vi "Test Control.vi"() -> ()   [LabVIEW 2012]
uses:
  2D Buffer Display.xctl
  <vilib>/Utility/miscctls.llb/LVBoundsTypeDef.ctl
  <vilib>/Utility/miscctls.llb/LVPositionTypeDef.ctl
panel:
  in  "Tab Control Pane Dimension":T1
  in  "Relative Size":dbl
  in  "Tab Control":enum32{"Page 1", "Page 2"}(tab)
  out "2D Buffer Display 3":cluster{"data_out":sgl[][], "time":timestamp}(xcontrol)
  out "2D Buffer Display 2":cluster{"data_out":sgl[][], "time":timestamp}(xcontrol)
  out "2D Buffer Display":cluster{"data_out":sgl[][], "time":timestamp}(xcontrol)
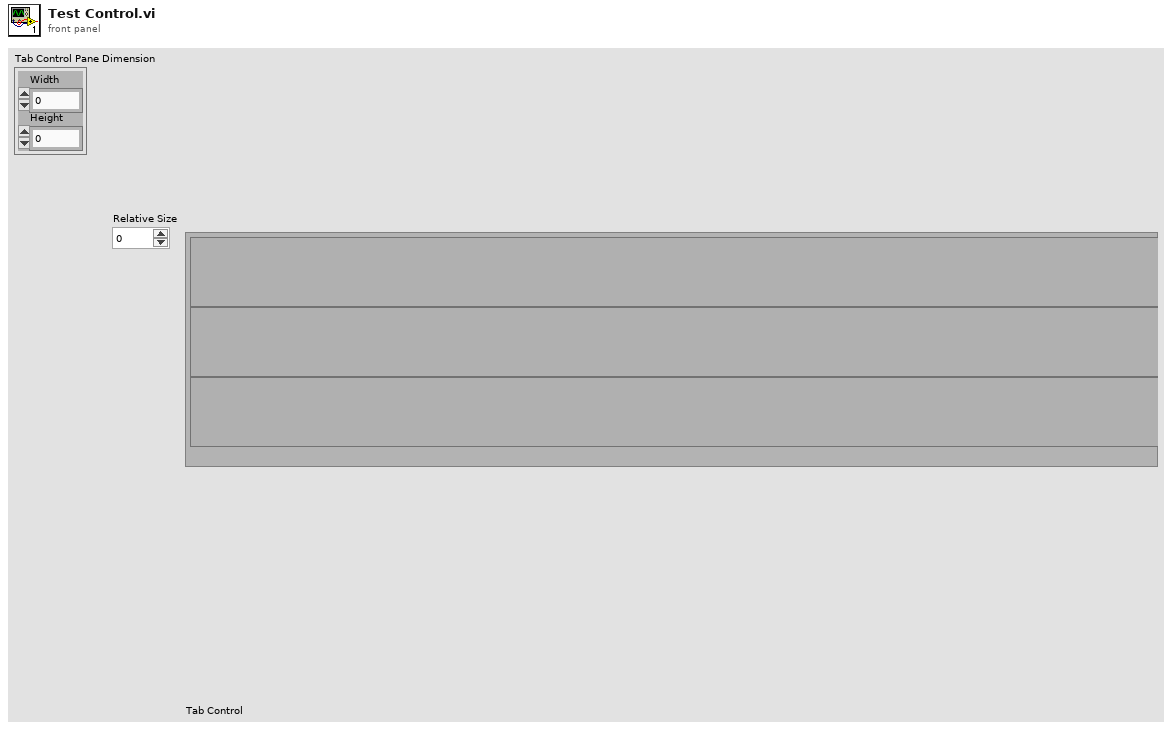
[diagram p1: front panel]
types:
  T1 = typedef "LVBoundsTypeDef.ctl" = cluster{"Width":u32, "Height":u32}
  T2 = typedef "LVPositionTypeDef.ctl" = cluster{"Left":i32, "Top":i32}
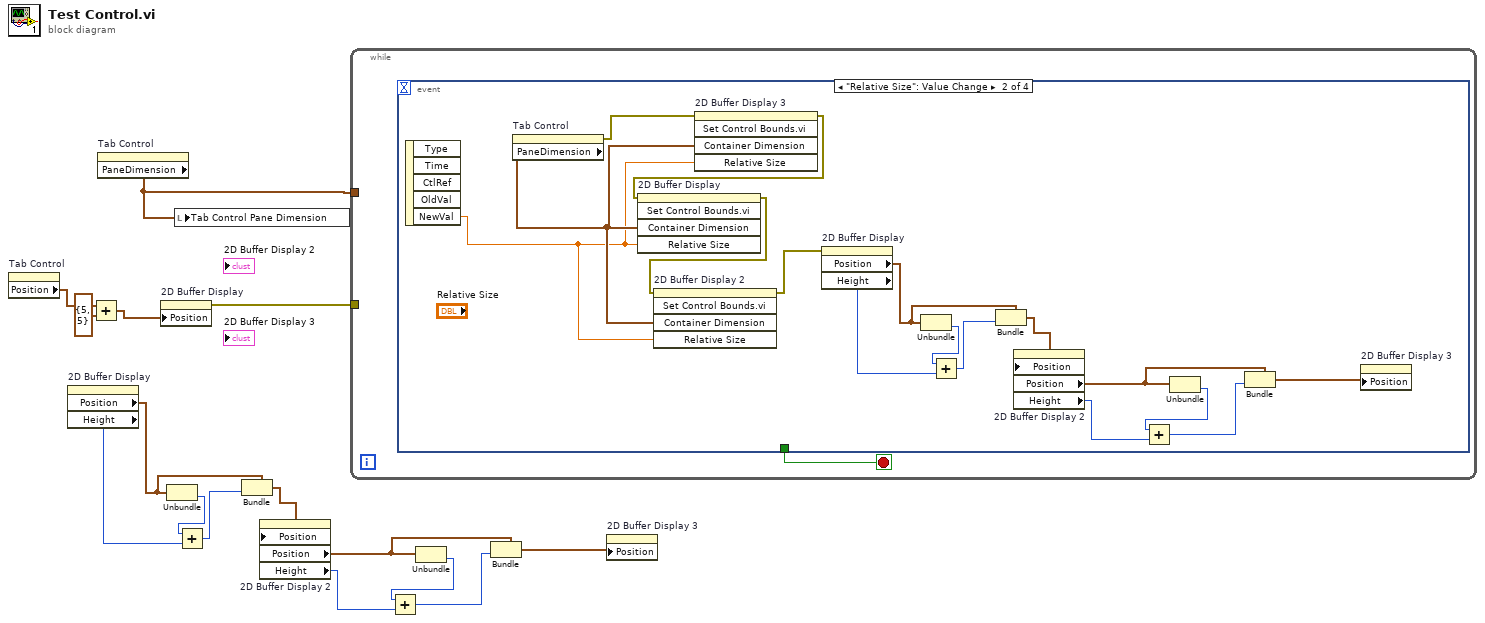
[diagram p0: block diagram]
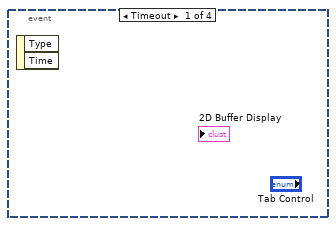
[diagram p2: hidden frame]
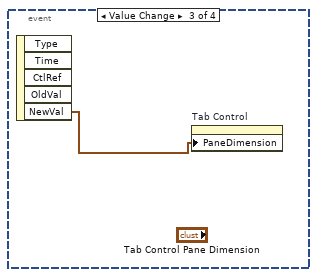
[diagram p3: hidden frame]
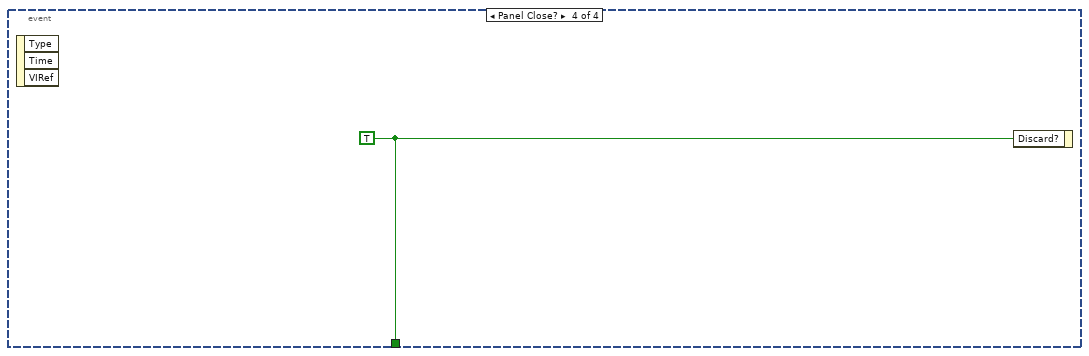
[diagram p4: hidden frame]
diagram:
  n1 = property on="Tab Control" class="TabCtl (strict)"() -> ("Position"=w14:T2)  [unwired: 2 in, 2 out]
  n2 = property on="2D Buffer Display" class="2D Buffer Display (strict)"() -> ("Position"=w7:T2, "Height"=w9:u32)  [unwired: 2 in, 2 out]
  n3 = Add(x=w14, y=T2 {"Left"=5, "Top"=5}) -> (x+y=w12:T2)
  n4 = property on="Tab Control" class="TabCtl (strict)"() -> ("PaneDimension"=w15:T1)  [unwired: 2 in, 2 out]
  n5 = property on="2D Buffer Display" class="2D Buffer Display (strict)"("Position"=w12) -> (error out=w11:errorcluster)  [unwired: 2 in, 1 out]
  n6 = Unbundle(w7) -> ("Top"=w10:i32)  [unwired: 1 out]
  n7 = local write "Tab Control Pane Dimension"(w15) -> ()
  n8 = Add(x=w10, y=w9) -> (x+y=w8:u32)
  n9 = Bundle(cluster=w7, "Top"=w8) -> (w6:T2)  [unwired: 1 in]
  n10 = property on="2D Buffer Display 2" class="2D Buffer Display (strict)"("Position"=w6) -> ("Position"=w5:T2, "Height"=w3:u32)  [unwired: 2 in, 2 out]
  n11 = while {
    tunnel: w15 -> [_]
    tunnel: w11 -> [_]
    stop <- w16 stop-if-true
    n12 = event shown="[1] \"Relative Size\": Value Change" {
      selector: _ -> [_ _ _ _]
      dyn-events: _ -> [_ _ _ _]
      timeout: _ -> [_ _ _ _]
      tunnel: [_ _ _ w34] -> w16
      event Timeout {
        n13 = event-data() -> ()  [unwired: 1 in, 2 out]
      }
      event "Relative Size": Value Change {
        n14 = event-data() -> ("NewVal"=w31:dbl)  [unwired: 1 in, 4 out]
        n15 = property on="Tab Control" class="TabCtl (strict)"() -> (error out=w20:errorcluster, "PaneDimension"=w32:T1)  [unwired: 2 in, 1 out]
        n16 = invoke on="2D Buffer Display 3" class="2D Buffer Display (strict)" method="Set Control Bounds.vi"(error in=w20, "Container Dimension"=w32, "Relative Size"=w31) -> (error out=w19:errorcluster)  [unwired: 2 in, 4 out]
        n17 = invoke on="2D Buffer Display" class="2D Buffer Display (strict)" method="Set Control Bounds.vi"(error in=w19, "Container Dimension"=w32, "Relative Size"=w31) -> (error out=w18:errorcluster)  [unwired: 2 in, 4 out]
        n18 = invoke on="2D Buffer Display 2" class="2D Buffer Display (strict)" method="Set Control Bounds.vi"(error in=w18, "Container Dimension"=w32, "Relative Size"=w31) -> (error out=w17:errorcluster)  [unwired: 2 in, 4 out]
        n19 = property on="2D Buffer Display" class="2D Buffer Display (strict)"(error in=w17) -> ("Position"=w24:T2, "Height"=w22:u32)  [unwired: 1 in, 2 out]
        n20 = Unbundle(w24) -> ("Top"=w21:i32)  [unwired: 1 out]
        n21 = Add(x=w21, y=w22) -> (x+y=w23:u32)
        n22 = Bundle(cluster=w24, "Top"=w23) -> (w25:T2)  [unwired: 1 in]
        n23 = property on="2D Buffer Display 2" class="2D Buffer Display (strict)"("Position"=w25) -> ("Position"=w26:T2, "Height"=w28:u32)  [unwired: 2 in, 2 out]
        n24 = Unbundle(w26) -> ("Top"=w27:i32)  [unwired: 1 out]
        n25 = Add(x=w27, y=w28) -> (x+y=w29:u32)
        n26 = Bundle(cluster=w26, "Top"=w29) -> (w30:T2)  [unwired: 1 in]
        n27 = property on="2D Buffer Display 3" class="2D Buffer Display (strict)"("Position"=w30) -> ()  [unwired: 2 in, 2 out]
      }
      event Value Change {
        n28 = event-data() -> ("NewVal"=w33:T1)  [unwired: 1 in, 4 out]
        n29 = property on="Tab Control" class="TabCtl (strict)"("PaneDimension"=w33) -> ()  [unwired: 2 in, 2 out]
      }
      event Panel Close? {
        w34 = TRUE ("Discard?")
        n30 = event-data() -> ()  [unwired: 1 in, 3 out]
        n31 = event-data("Discard?"=w34) -> ()  [unwired: 1 in, 1 out]
      }
    }
  }
  n32 = Unbundle(w5) -> ("Top"=w4:i32)  [unwired: 1 out]
  n33 = Add(x=w4, y=w3) -> (x+y=w2:u32)
  n34 = Bundle(cluster=w5, "Top"=w2) -> (w1:T2)  [unwired: 1 in]
  n35 = property on="2D Buffer Display 3" class="2D Buffer Display (strict)"("Position"=w1) -> ()  [unwired: 2 in, 2 out]
